vi "FFT_Python.vi"() -> ()   [LabVIEW 2020]
uses:
  <vilib>/measure/NI_MABase.lvlib
panel:
  out "FFT 2":waveform(dbl)(graph)
  out "FFT":dbl[](graph)
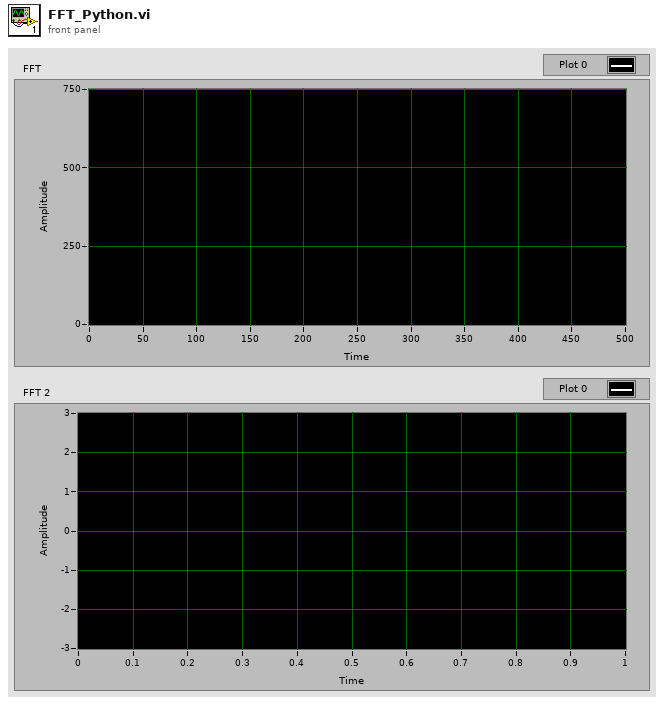
[diagram p1: front panel]
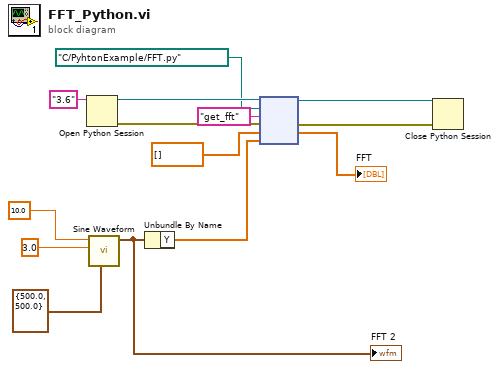
[diagram p0: block diagram]
diagram:
  n1 = Open Python Session(python version="3.6" ("Python version")) -> (session out=w14:refnum<k35>, error out=w13:errorcluster)  [unwired: 2 in]
  n2 = call <vilib>:"Sine Waveform.vi"("sampling info"=cluster{"Fs":dbl, "#s":dbl} {"Fs"=500.0, "#s"=500.0}, "amplitude"=3.0, "frequency"=10.0) -> ("signal out"=w2:waveform(dbl))  [unwired: 7 in, 1 out]
  "FFT 2" <- w2
  n3 = Unbundle By Name(w2) -> ("Y"=w5:dbl[])
  n4 = node(w14, path "C:/PyhtonExample/FFT.py" ("module path"), "get_fft" ("function name"), w13, dbl[] [], w5) -> (w12:refnum<k35>, w11:errorcluster, →"FFT":dbl[])  [unwired: 1 in, 2 out]
  n5 = Close Python Session(session in=w12, error in=w11) -> ()  [unwired: 1 out]
